vi "UDP Server Subnet C.vi"(8 "error in (no error)":errorcluster, 9 "Subnet":string, 10 "User Event in":refnum<class "User Event.lvclass">, 11 "UDP Port":u16=5005) -> (0 "error out":errorcluster, 2 "Array":u8[](array[numeric]), 3 "Output":string)   [LabVIEW 2016]
uses:
  User Events/User Event.lvclass
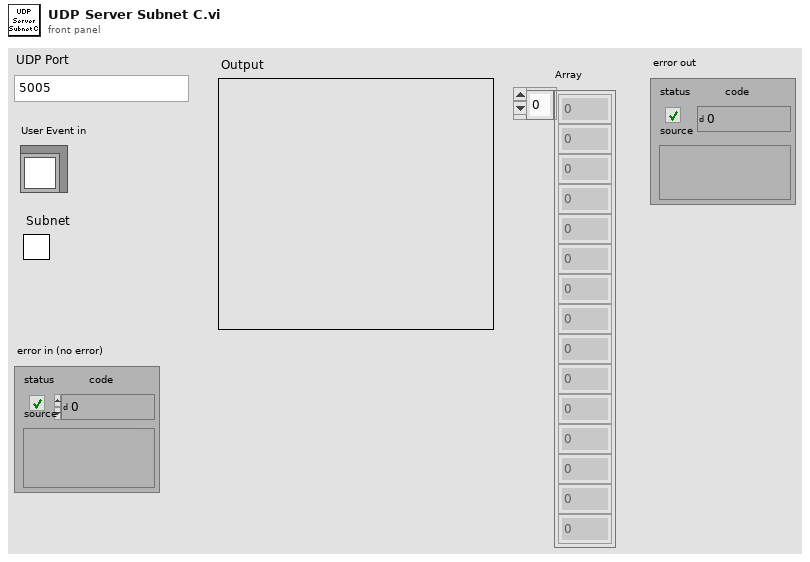
[diagram p1: front panel]
types:
  T1 = typedef "M1M3SupSimUserEvents.ctl" = cluster{"ILCResponse":refnum<user-event>, "StopUDPServer":refnum<user-event>}
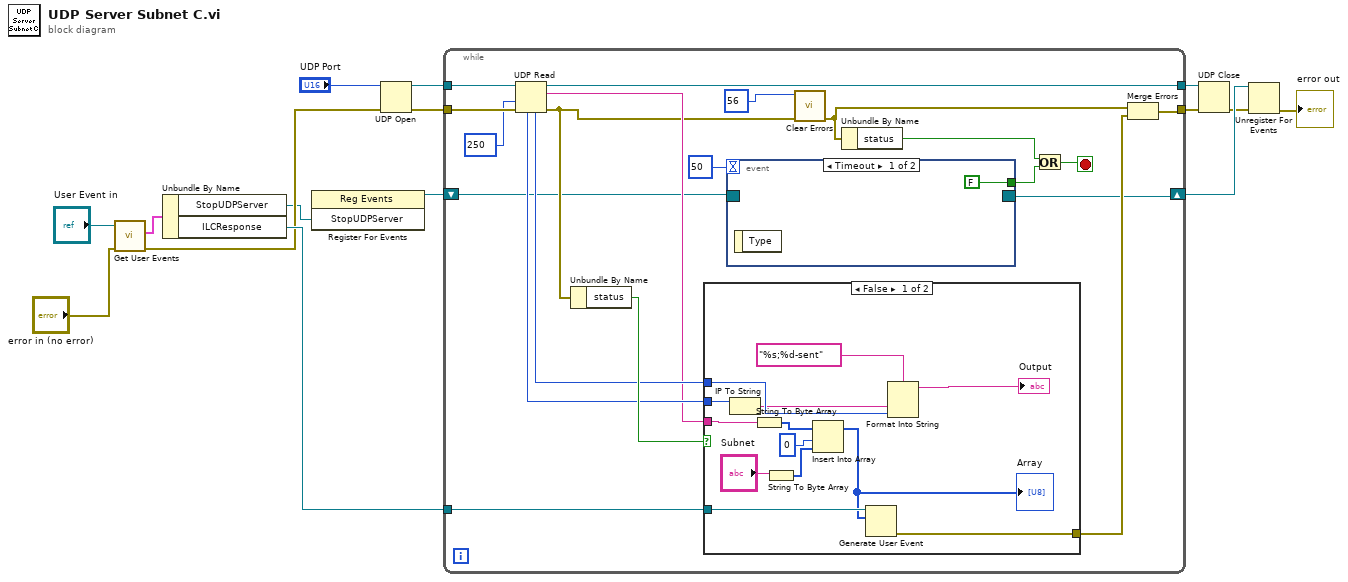
[diagram p0: block diagram]
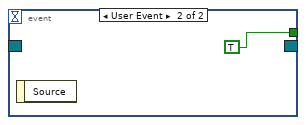
[diagram p2: hidden frame]
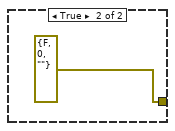
[diagram p3: hidden frame]
diagram:
  n1 = call "Get User Events.vi"("error in (no error)"="error in (no error)", "User Event in"="User Event in") -> ("error out"=w14:errorcluster, "User Events"=w11:T1)  [unwired: 7 in, 1 out]
  n2 = Unbundle By Name(w11) -> ("StopUDPServer"=w12:refnum<user-event>, "ILCResponse"=w15:refnum<user-event>)
  n3 = register-events(w12) -> (reference out=w6:refnum<event-registration>)  [unwired: 2 in, 1 out]
  n4 = UDP Open(8:w14, 11:"UDP Port") -> (port=w2:refnum<k16>, 0:w3:errorcluster)  [unwired: 3 in, 1 out]
  n5 = while {
    tunnel: w2 -> [w35]
    tunnel: w3 -> [w34]
    tunnel: [w22] -> w5
    tunnel: [w32] -> w4
    shift-right: [w17] -> w8
    shift-left: w6 -> [w20]
    tunnel: w15 -> [w16]
    stop <- w21 stop-if-true
    n6 = UDP Read(connection ID=w35, timeout ms (25000)=250, 8:w34) -> (data out=w28:string, error out=w27:errorcluster, 3:w32:refnum<k16>, 4:w29:u16, 6:w30:u32)  [unwired: 1 in]
    n7 = Unbundle By Name(w27) -> ("status"=w31:bool)
    n8 = case shown="False" w31 {
      tunnel: w30 -> [w50 _]
      tunnel: w29 -> [w49 _]
      tunnel: w28 -> [w46 _]
      tunnel: [w44 errorcluster {"status"=FALSE, "code"=0, "source"=""} ("error out")] -> w23
      tunnel: w16 -> [w45 _]
      frame False {
        n9 = IP To String(2:w50) -> (0:w47:string)  [unwired: 1 in]
        n10 = String To Byte Array(string=w46) -> (unsigned byte array=w40:u8[])
        n11 = String To Byte Array(string="Subnet") -> (unsigned byte array=w39:u8[])
        n12 = Insert Into Array(array=w40, index=0, new element=w39) -> (w41:u8[])
        "Array" <- w41
        n13 = Generate User Event(user event=w45, event data cluster=w41) -> (error out=w44:errorcluster)  [unwired: 2 in, 1 out]
        n14 = Format Into String(format string="%s;%d-sent", w47, w49) -> (resulting string=→"Output":string)  [unwired: 2 in, 1 out]
      }
      frame True {
      }
    }
    n15 = event shown="[0] Timeout" {
      selector: w20 -> [_ _]
      dyn-events: [_ _] -> w17
      timeout: 50 -> [_ _]
      tunnel: [FALSE TRUE] -> w18
      event Timeout {
        n16 = event-data() -> ()  [unwired: 1 in, 1 out]
      }
      event User Event {
        n17 = event-data() -> ()  [unwired: 1 in, 1 out]
      }
    }
    n18 = call <vilib>:"Clear Errors.vi"("error in (no error)"=w27, "specific error code to clear (0: all)"=56) -> ("error out"=w24:errorcluster)  [unwired: 4 in, 1 out]
    n19 = Unbundle By Name(w24) -> ("status"=w25:bool)
    n20 = Or(x=w25, y=w18) -> (x .or. y?=w21:bool)
    n21 = Merge Errors(w24, w23) -> (w22:errorcluster)
  }
  n22 = UDP Close(connection ID=w4, 8:w5) -> (error out=w7:errorcluster)  [unwired: 1 out]
  n23 = Unregister For Events(event registration refnum=w8, error in=w7) -> (error out=→"error out":errorcluster)
